vi "check trigger.vi"(7 "Edge Direction":T1, 9 "No trigger?":bool, 10 "triggerchannel index":i32, 11 "data table in":T2) -> (2 "Trigger":bool, 3 "Data table out":T2)   [LabVIEW 2013, in "TDMS datalogger runtime.lvclass"]
uses:
  TDMS datalogger runtime.lvclass
  <vilib>/NI/Tag Bus/table/data table.ctl
  configuration/Edge Direction.ctl
  <vilib>/NI/Tag Bus/table/data polymorphs/read one/read Boolean.vi
  <vilib>/NI/Tag Bus/table/data table.lvlib
  configuration/TDMS datalogger configuration.lvclass
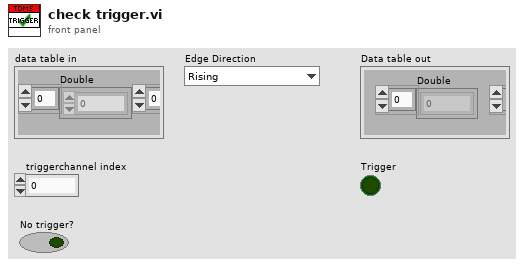
[diagram p1: front panel]
types:
  T1 = typedef "TDMS datalogger configuration.lvclass/Edge Direction.ctl" = enum16{"Rising", "Falling"}
  T2 = typedef "tag bus.lvlib/data table.lvlib/data table.ctl" = cluster{"Double":dbl[], "Single":sgl[], "I64":i64[], "I32":i32[], "I16":i16[], "I8":i8[], "U64":u64[], "U32":u32[], "U16":u16[], "U8":u8[], "Boolean":bool[], "String":string[], "Array of Double":cluster{"DBL Array":dbl[]}[], "Array of Single":cluster{"SGL Array":sgl[]}[], "Array of I64":cluster{"I64 Array":i64[]}[], "Array of I32":cluster{"I32 Array":i32[]}[], "Array of I16":cluster{"I16 Array":i16[]}[], "Array of I8":cluster{"I8 Array":i8[]}[], "Array of U64":cluster{"U64 Array":u64[]}[], "Array of U32":cluster{"U32 Array":u32[]}[], "Array of U16":cluster{"U16 Array":u16[]}[], "Array of U8":cluster{"U8 Array":u8[]}[], "Array of Boolean":cluster{"Boolean Array":bool[]}[], "Array of String":cluster{"String Array":string[]}[]}
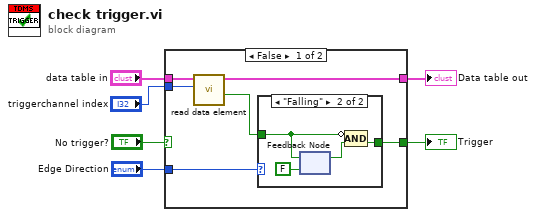
[diagram p0: block diagram]
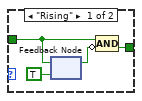
[diagram p2: hidden frame]
diagram:
  n1 = case shown="False" "No trigger?" {
    selector: "No trigger?" -> [_ w22]
    tunnel: "triggerchannel index" -> [w12 _]
    tunnel: [w11 w21] -> w5
    tunnel: "data table in" -> [w10 w21]
    tunnel: [w9 w22] -> w3
    tunnel: "Edge Direction" -> [w7 _]
    frame False {
      n2 = call-poly <vilib>:"read data element.vi"("index"=w12, "data table in"=w10) -> ("value"=w8:bool, "data table out"=w11:T2)  [unwired: 8 in]
      n3 = case shown="\"Falling\"" w7 {
        tunnel: w8 -> [w16 w17]
        tunnel: [w13 w19] -> w9
        frame "Rising" {
          n4 = feedback #1(TRUE ("Trigger")) -> (w15:bool)
          n5 = feedback-in #1(w16) -> ()
          n6 = Compound Arithmetic op=AND(w16, invert w15) -> (w13:bool)
        }
        frame "Falling" {
          n7 = feedback #2(FALSE ("Trigger")) -> (w18:bool)
          n8 = feedback-in #2(w17) -> ()
          n9 = Compound Arithmetic op=AND(invert w17, w18) -> (w19:bool)
        }
      }
    }
    frame True {
    }
  }
  "Data table out" <- w5
  "Trigger" <- w3
